vi "SupervisorySystem.vi"() -> ()   [LabVIEW 2025]
panel:
  out "AgitatorSystem/AgitatorState":string caption="Mode"
  # "SUPERVISORY"
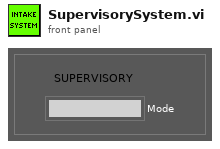
[diagram p1: front panel]
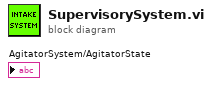
[diagram p0: block diagram]
diagram:
